vi "Practica 10 - Cadenas.vi"() -> ()   [LabVIEW 2023]
panel:
  out "substring":string
  in  "Length (rest)":i32=2
  in  "Offset (0)":i32=1
  out "Número de caracteres":i32
  out "Display de cadena":string
  in  "Control de cadena":string
  # "ACTIVIDAD CADENAS"
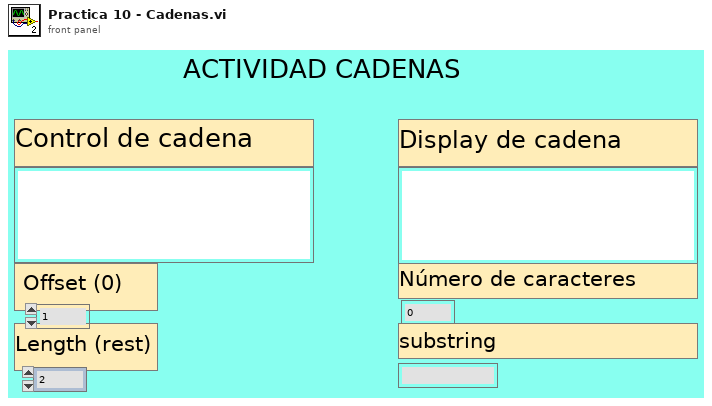
[diagram p1: front panel]
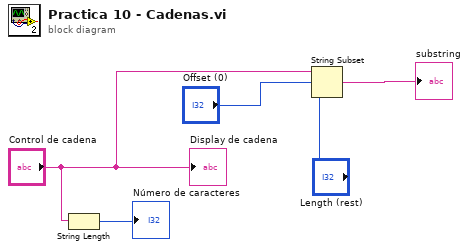
[diagram p0: block diagram]
diagram:
  n1 = String Length(string="Control de cadena") -> (length=→"Número de caracteres":i32)
  n2 = String Subset(string="Control de cadena", offset (0)="Offset (0)", length (rest)="Length (rest)") -> (substring=→"substring":string)
  "Display de cadena" <- "Control de cadena"
